vi "Create Sysdef Hardware Tree.vi"(5 "Create bank channels":bool, 6 "Default Value":dbl, 7 "temp param":T2={"A"=0.00139999995008111, "B"=0.00023700000019744039, "C"=9.899999753315569e-08, "R0"=1000.0}, 8 "Error In":errorcluster, 9 "Mode":T3, 10 "number of channels":i32, 11 "Section Refs":T1[](array[typedef]) format="%.0x") -> (0 "Error Out":errorcluster)   [LabVIEW 2023, in "NI 272x Resistive Simulation Custom Device Configuration.lvlib"]
doc: "Reconfigure veristand channels based on device selected."
uses:
  NI 272x Resistive Simulation Custom Device Configuration.lvlib
  Controls/Channel Mode.ctl
  <instrlib>/ni272xReferenceVIs/ni272xReferenceVIs.llb/ni272x Callendar-Van Dusen RTD Parameters.ctl
  <vilib>/NI VeriStand/Custom Device API/Custom Device Item Ref.ctl
  <vilib>/NI VeriStand/Custom Device API/Custom Device Channel.ctl
  <vilib>/NI VeriStand/Custom Device API/Custom Device Channel Type.ctl
  Globals/Names.vi
  <vilib>/NI VeriStand/Custom Device API/Set Item Property (I32).vi
  <vilib>/NI VeriStand/Custom Device API/Set Item Property (U16).vi
  NI 272x Resistive Simulation Custom Device Shared.lvlib
  <vilib>/NI VeriStand/Custom Device API/Custom Device API.lvlib
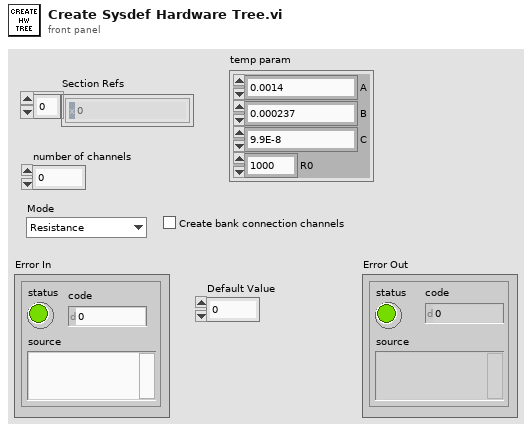
[diagram p1: front panel]
types:
  T1 = typedef "Custom Device API.lvlib/Custom Device Item Ref.ctl" = u64
  T2 = typedef "ni272x Callendar-Van Dusen RTD Parameters.ctl" = cluster{"A":dbl, "B":dbl, "C":dbl, "R0":dbl}
  T3 = typedef "NI 272x Resistive Simulation Custom Device Shared.lvlib/Channel Mode.ctl" = enum16{"Resistance", "RTD Temperature"}
  T4 = typedef "Custom Device API.lvlib/Custom Device Channel.ctl" = cluster{"Type":T5, "Units":string, "Default Value":dbl, "Faultable":bool, "Scalable":bool}
  T5 = typedef "Custom Device API.lvlib/Custom Device Channel Type.ctl" = enum16{"Input", "Output"}
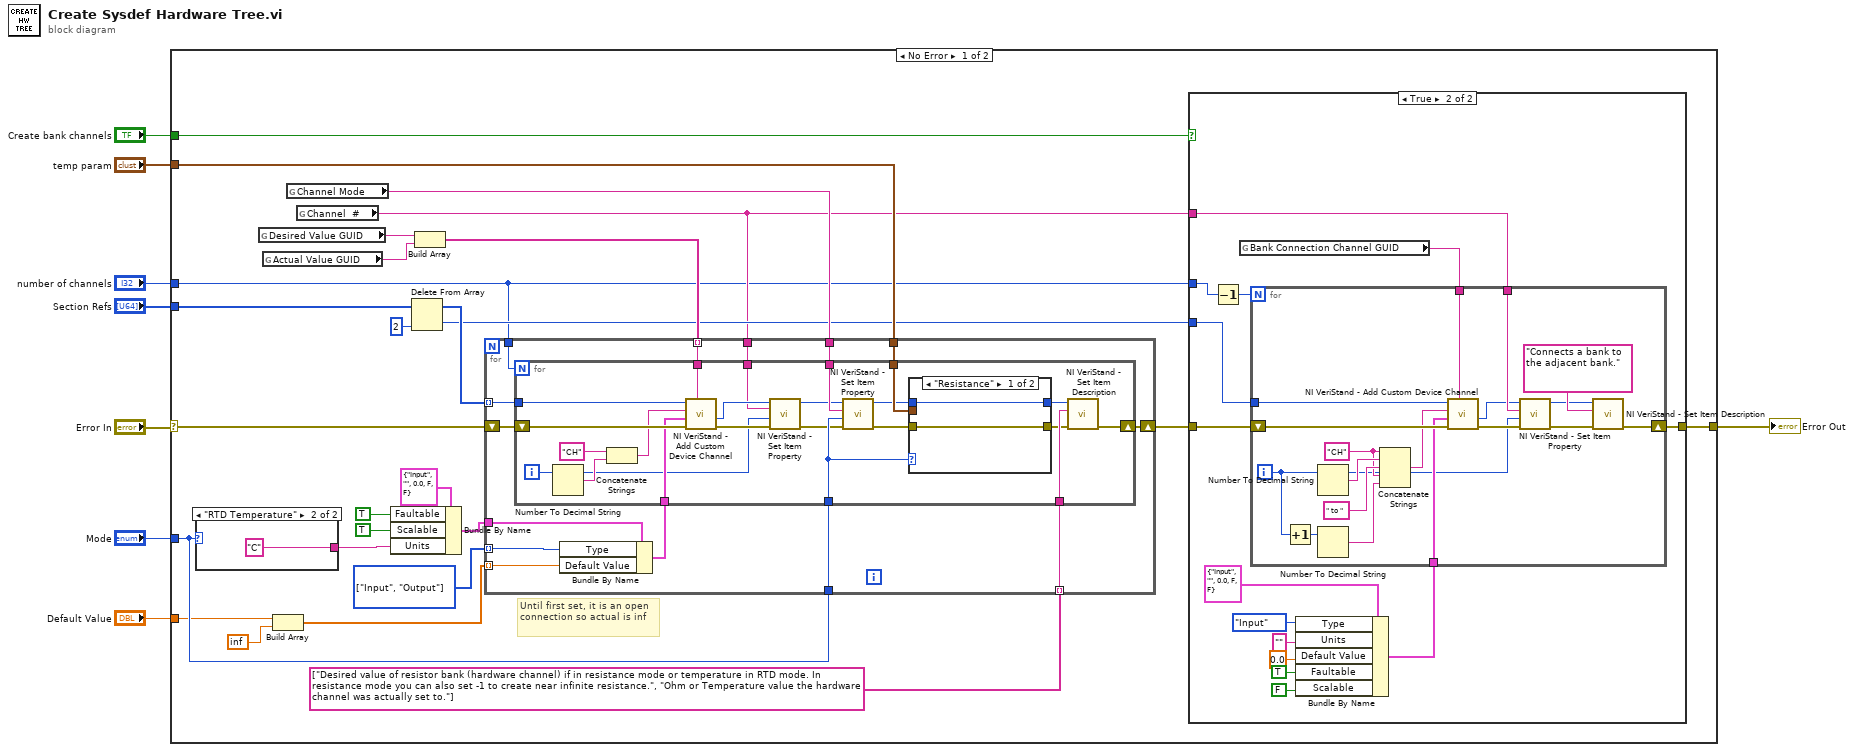
[diagram p0: block diagram]
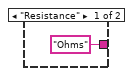
[diagram p3: hidden frame]
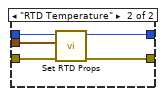
[diagram p4: hidden frame]
diagram:
  n1 = case shown="No Error" "Error In" {
    selector: "Error In" -> [w13 w113]
    tunnel: [w15 w113] -> w8
    tunnel: "Mode" -> [w25 _]
    tunnel: "number of channels" -> [w14 _]
    tunnel: "temp param" -> [w23 _]
    tunnel: "Create bank channels" -> [w21 _]
    tunnel: "Section Refs" -> [w12 _]
    tunnel: "Default Value" -> [w11 _]
    frame No Error {
      w17 = T5[] [enum."Input", enum."Output"] items=["Input", "Output"]
      # "Until first set, it is an open connection so actual is inf"
      n2 = case shown="\"RTD Temperature\"" w25 {
        tunnel: ["Ohms" ("Units") "C" ("Units")] -> w18
        frame "Resistance" {
        }
        frame "RTD Temperature" {
        }
      }
      n3 = global read "Names.vi" "Desired Value GUID"() -> (w32:string)
      n4 = global read "Names.vi" "Actual Value GUID"() -> (w31:string)
      n5 = Build Array(w11, inf) -> (w9:dbl[])
      n6 = global read "Names.vi" "Channel Mode"() -> (w24:string)
      n7 = global read "Names.vi" "Channel  #"() -> (w16:string)
      n8 = Bundle By Name(cluster=T4 {"Type"=enum."Input", "Units"="", "Default Value"=0.0, "Faultable"=FALSE, "Scalable"=FALSE} ("Channel"), "Faultable"=TRUE, "Scalable"=TRUE, "Units"=w18) -> (w26:T4)
      n9 = Delete From Array(array=w12, index=2) -> (deleted portion=w19:T1, array with subset deleted=w33:T1[])  [unwired: 1 in]
      n10 = Build Array(w32, w31) -> (w30:string[])
      n11 = for {
        tunnel: w33 -> [w82] mode=indexing
        shift-right: [w81] -> w20
        shift-left: w13 -> [w83]
        tunnel: w30 -> [w80] mode=indexing
        tunnel: w26 -> [w74]
        tunnel: w25 -> [w79]
        tunnel: w24 -> [w78]
        tunnel: w23 -> [w77]
        tunnel: string[] ["Desired value of resistor bank (hardware channel) if in resistance mode or temperature in RTD mode. In resistance mode you can also set -1 to create near infinite resistance.", "Ohm or Temperature value the hardware channel was actually set to."] -> [w76] mode=indexing
        tunnel: w16 -> [w75]
        tunnel: w17 -> [w72] mode=indexing
        tunnel: w14 -> [w71]
        tunnel: w9 -> [w70] mode=indexing
        n12 = Bundle By Name(cluster=w74, "Type"=w72, "Default Value"=w70) -> (w73:T4)
        n13 = for {
          N: w71 -> [_]
          tunnel: w82 -> [w104]
          shift-right: [w94] -> w81
          shift-left: w83 -> [w105]
          tunnel: w80 -> [w103]
          tunnel: w73 -> [w99]
          tunnel: w79 -> [w96]
          tunnel: w78 -> [w97]
          tunnel: w77 -> [w95]
          tunnel: w76 -> [w93]
          tunnel: w75 -> [w91]
          i -> [w90]
          n14 = Number To Decimal String(number=w90) -> (decimal integer string=w101:string)  [unwired: 1 in]
          n15 = Concatenate Strings("CH", w101) -> (w100:string)
          n16 = call <vilib>:"NI VeriStand - Add Custom Device Channel.vi"("GUID (Default Channel)"=w103, "error in (no error)"=w105, "Channel"=w99, "Channel Name"=w100, "Parent Ref in"=w104) -> ("error out"=w98:errorcluster, "Channel Ref"=w92:T1)  [unwired: 3 in, 2 out]
          n17 = call-poly <vilib>:"NI VeriStand - Set Item Property.vi"("error in (no error)"=w98, "Value"=w90, "Property Name"=w91, "Item Ref in"=w92) -> ("error out"=w85:errorcluster, "Item Ref out"=w84:T1)  [unwired: 5 in, 1 out]
          n18 = call-poly <vilib>:"NI VeriStand - Set Item Property.vi"("error in (no error)"=w85, "Value"=w96, "Property Name"=w97, "Item Ref in"=w84) -> ("error out"=w89:errorcluster, "Item Ref out"=w88:T1)  [unwired: 5 in, 1 out]
          n19 = case shown="\"Resistance\"" w96 {
            tunnel: w89 -> [w106 w112]
            tunnel: w88 -> [w107 w111]
            tunnel: [w107 w110] -> w87
            tunnel: [w106 w109] -> w86
            tunnel: w95 -> [_ w108]
            frame "Resistance" {
            }
            frame "RTD Temperature" {
              n20 = call "Set RTD Props.vi"("error in (no error)"=w112, "temp param"=w108, "Item Ref in"=w111) -> ("error out"=w109:errorcluster, "Item Ref out"=w110:T1)  [unwired: 7 in]
            }
          }
          n21 = call <vilib>:"NI VeriStand - Set Item Description.vi"("error in (no error)"=w86, "Description"=w93, "Item Ref in"=w87) -> ("error out"=w94:errorcluster)  [unwired: 6 in, 2 out]
        }
      }
      n22 = case shown="True" w21 {
        tunnel: w20 -> [w35 w48]
        tunnel: w19 -> [_ w46]
        tunnel: w14 -> [_ w49]
        tunnel: w16 -> [_ w38]
        tunnel: [w35 w37] -> w15
        frame False {
        }
        frame True {
          n23 = Decrement(x=w49) -> (x-1=w47:i32)
          n24 = global read "Names.vi" "Bank Connection Channel GUID"() -> (w36:string)
          n25 = Bundle By Name(cluster=T4 {"Type"=enum."Input", "Units"="", "Default Value"=0.0, "Faultable"=FALSE, "Scalable"=FALSE} ("Channel"), "Type"=Custom_Device_Channel_Type."Input", "Units"="", "Default Value"=0.0, "Faultable"=TRUE, "Scalable"=FALSE) -> (w39:T4)
          n26 = for {
            N: w47 -> [_]
            shift-right: [w57] -> w37
            shift-left: w48 -> [w67]
            tunnel: w46 -> [w66]
            tunnel: w39 -> [w59]
            tunnel: w38 -> [w56]
            tunnel: w36 -> [w53]
            i -> [w55]
            w62 = "CH"
            n27 = Increment(x=w55) -> (x+1=w64:i32)
            n28 = Number To Decimal String(number=w55) -> (decimal integer string=w65:string)  [unwired: 1 in]
            n29 = Number To Decimal String(number=w64) -> (decimal integer string=w61:string)  [unwired: 1 in]
            n30 = Concatenate Strings(w62, w65, " to ", w62, w61) -> (w60:string)
            n31 = call <vilib>:"NI VeriStand - Add Custom Device Channel.vi"("GUID (Default Channel)"=w53, "error in (no error)"=w67, "Channel"=w59, "Channel Name"=w60, "Parent Ref in"=w66) -> ("error out"=w58:errorcluster, "Channel Ref"=w54:T1)  [unwired: 3 in, 2 out]
            n32 = call-poly <vilib>:"NI VeriStand - Set Item Property.vi"("error in (no error)"=w58, "Value"=w55, "Property Name"=w56, "Item Ref in"=w54) -> ("error out"=w51:errorcluster, "Item Ref out"=w50:T1)  [unwired: 5 in, 1 out]
            n33 = call <vilib>:"NI VeriStand - Set Item Description.vi"("error in (no error)"=w51, "Description"="Connects a bank to the adjacent bank.", "Item Ref in"=w50) -> ("error out"=w57:errorcluster)  [unwired: 6 in, 2 out]
          }
        }
      }
    }
    frame Error {
    }
  }
  "Error Out" <- w8
